vi "Export ECAT Section to XML.vi"() -> ()   [LabVIEW 2015, in "Scan Engine Custom Device.lvlib"]
uses:
  Scan Engine Custom Device.lvlib
  <vilib>/xml/Close Reference(Node).vi
  <vilib>/xml/NI_XML.lvlib
  <resource>/objmgr/DOMUserDefRef.rc
panel:
  in  "input 1":string="EK1100 EtherCAT Coupler (2A E-Bus)"
  out "size(s)":i32
  out "Array":string[](array[string])
  out "error out":errorcluster
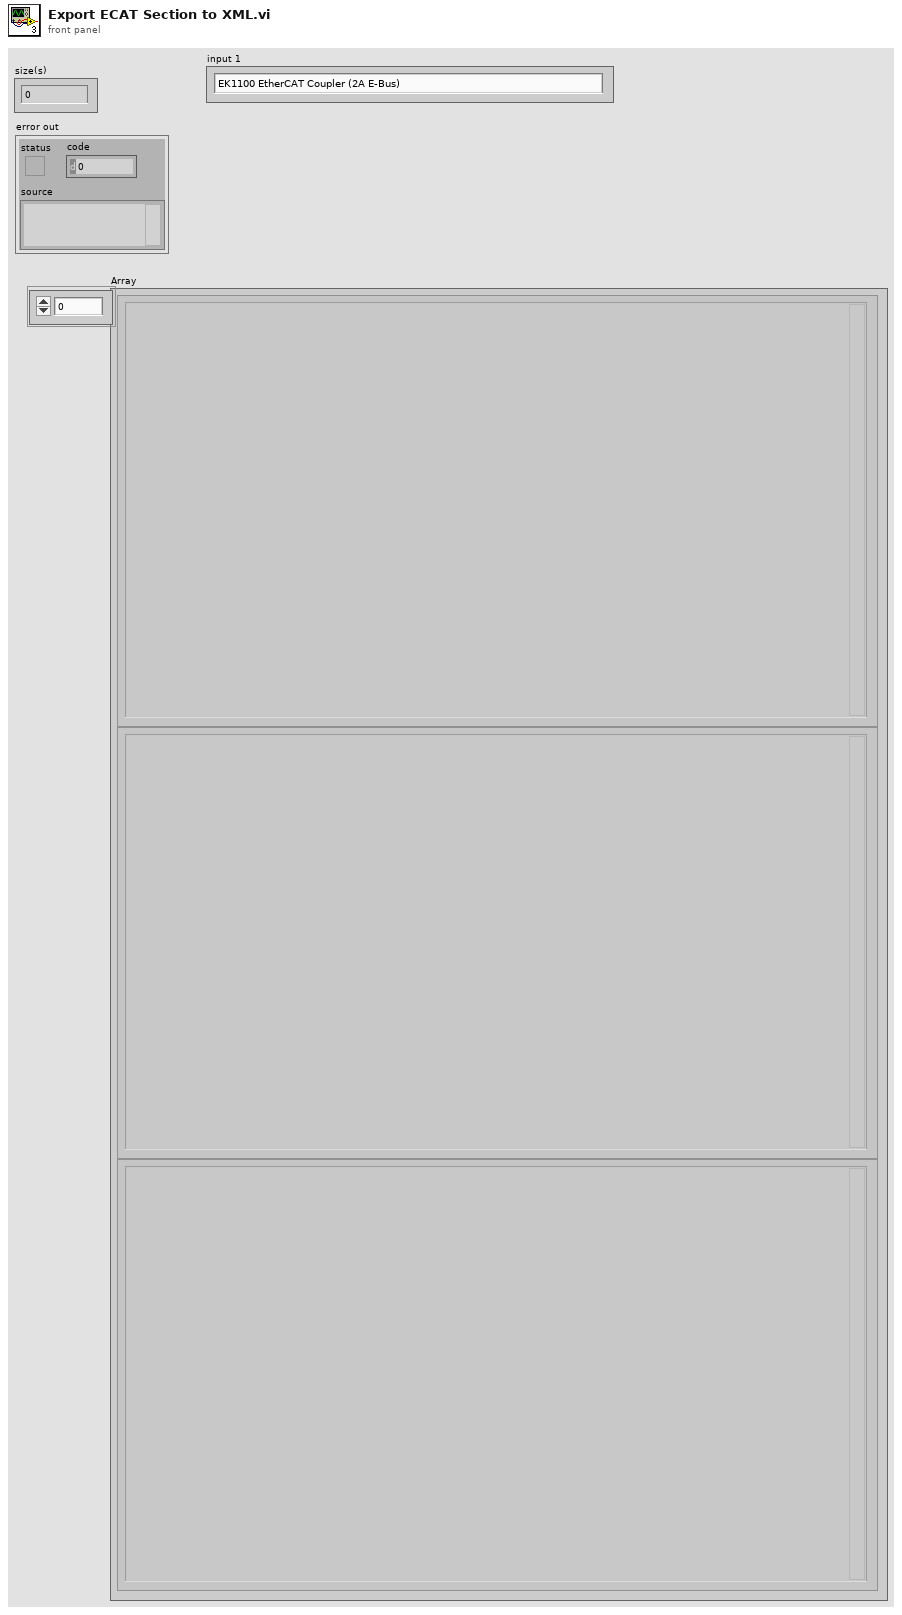
[diagram p1: front panel]
types:
  T1 = enum16{"open", "replace", "create", "open or create", "replace or create", "replace or create with confirmation"}
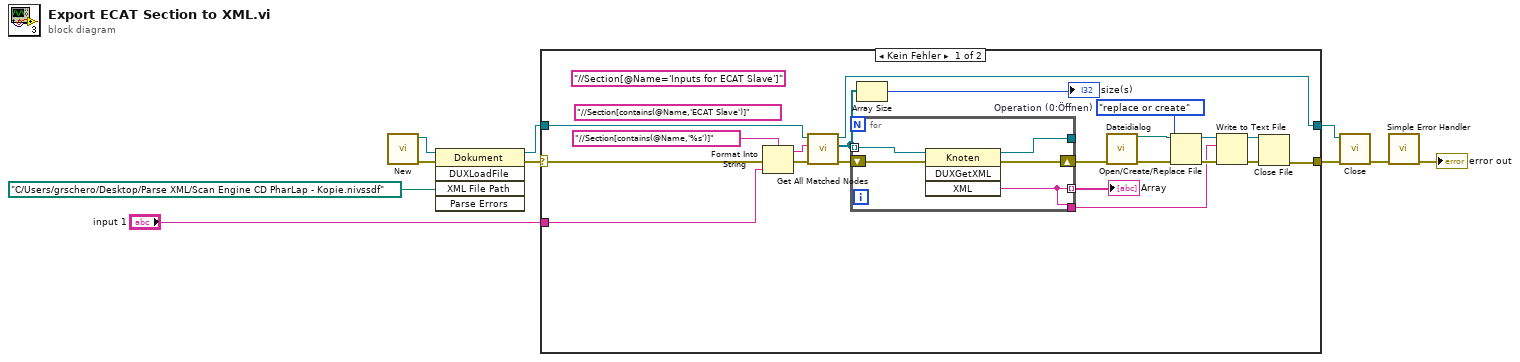
[diagram p0: block diagram]
diagram:
  n1 = call <vilib>:"New.vi"() -> ("error out"=w8:errorcluster, "DOM document out"=w9:refnum<k20>)  [unwired: 8 in]
  n2 = invoke class="Dokument" method="DUXLoadFile"(reference=w9, error in=w8, "XML File Path"=path "C:/Users/grschero/Desktop/Parse XML/Scan Engine CD PharLap - Kopie.nivssdf") -> (reference out=w7:refnum<k20>, error out=w4:errorcluster)  [unwired: 2 in, 3 out]
  n3 = case shown="Kein Fehler" w4 {
    selector: w4 -> [w23 w37]
    tunnel: w7 -> [w20 w38]
    tunnel: [w31 w38] -> w6
    tunnel: [w12 w37] -> w5
    tunnel: "input 1" -> [w25 _]
    frame No Error {
      w17 = T1."replace or create"  # Operation (0:Öffnen)
      (unwired) "//Section[contains(@Name,'ECAT Slave')]" ("XPath expression")
      (unwired) "//Section[@Name='Inputs for ECAT Slave']" ("XPath expression")
      n4 = Format Into String(format string="//Section[contains(@Name,'%s')]" ("XPath expression"), error in=w23, w25) -> (resulting string=w24:string, error out=w22:errorcluster)  [unwired: 1 in]
      n5 = call <vilib>:"Get All Matched Nodes.vi"("error in (no error)"=w22, "XPath expression"=w24, "node in"=w20) -> ("error out"=w30:errorcluster, "node result array"=w29:refnum<k20>[], "node out"=w31:refnum<k20>)  [unwired: 6 in]
      n6 = for {
        tunnel: w29 -> [w36] mode=indexing
        shift-right: [w34] -> w21
        shift-left: w30 -> [w35]
        tunnel: [w32] -> w27 mode=indexing
        tunnel: [w33] -> _
        tunnel: [w32] -> w11
        n7 = invoke class="Knoten" method="DUXGetXML"(reference=w36, error in=w35) -> (reference out=w33:refnum<k20>, error out=w34:errorcluster, "XML"=w32:string)  [unwired: 2 in, 1 out]
      }
      "Array" <- w27
      n8 = Array Size(array=w29) -> (size(s)=→"size(s)":i32)
      n9 = call "Dateidialog"("error in"=w21) -> ("selected path"=w18:path, "error out"=w16:errorcluster)  [unwired: 11 in, 2 out]
      n10 = Open/Create/Replace File(file path (use dialog)=w18, error in=w16, operation (0:open)=w17) -> (refnum out=w19:refnum<file>, error out=w15:errorcluster)  [unwired: 3 in, 1 out]
      n11 = Write to Text File(file (use dialog)=w19, text=w11, error in=w15) -> (refnum out=w13:refnum<file>, error out=w14:errorcluster)  [unwired: 1 in, 1 out]
      n12 = Close File(refnum=w13, error in=w14) -> (error out=w12:errorcluster)  [unwired: 1 out]
    }
    frame Error {
    }
  }
  n13 = call-poly <vilib>:"Close.vi"("error in (no error)"=w5, "node"=w6) -> ("error out"=w10:errorcluster)  [unwired: 7 out]
  n14 = call <vilib>:"Simple Error Handler.vi"("error in (no error)"=w10) -> ("error out"=→"error out":errorcluster)  [unwired: 4 in, 4 out]
